vi "canDataSort.vi"() -> ()   [LabVIEW 2023] (continued)
      2032  1FFFFFFF   00000004    8        00\t00\tFF\tFF\tFF\tFF\tFF\tFF\r\n      2023  0CF102A7   00000004    8        30\t75\tE0\t2E\t80\tFF\tFF\tFD\r\n      2023  0CF101A7   00000004    8        68\t00\t97\tCC\t00\t16\t39\t7F\r\n      2046  18F121F0   00000004    8        09\t19\t00\t00\tFF\tFF\tB0\t01\r\n      2045  18F106A7   00000004    8        00\tF7\tFF\tFF\tFF\tFF\tFF\t99\r\n      2045  0CF104A7   00000004    8        F0\t60\t22\tFC\tFF\tFF\tFF\t4C\r\n      2044  0CF103A7   00000004    8        17\t1F\t08\t60\tB1\t1F\t08\t4C\r\n      2044  0CF102A7   00000004    8        30\t75\tE0\t2E\t80\tFF\tFF\tFD\r\n      2043  0C3C4D4A   00000004    8        BE\tFF\tFF\t7F\t18\tFF\tFF\t4C\r\n      2043  0CF101A7   00000004    8        68\t00\t97\tCC\t00\t16\t39\t80\r\n      2042  18F120F0   00000004    8        2B\t75\t60\tB1\tB0\t01\tFF\tFF\r\n      2041  18F11FF0   00000004    8        FF\t3F\t90\t68\t88\t1B\t10\tCC\r\n      2032  1FFFFFFF   00000004    8        00\t00\tFF\tFF\tFF\tFF\tFF\tFF\r\n      2023  0CF102A7   00000004    8        30\t75\tE0\t2E\t80\tFF\tFF\tFD\r\n      2047  1FFFFFFF   00000004    8        00\t00\tFF\tFF\tFF\tFF\tFF\tFF\r\n      2046  18F121F0   00000004    8        09\t19\t00\t00\tFF\tFF\tB0\t01\r\n      2045  18F106A7   00000004    8        00\tF7\tFF\tFF\tFF\tFF\tFF\t99\r\n      2045  0CF104A7   00000004    8        F0\t60\t22\tFC\tFF\tFF\tFF\t4C\r\n      2044  0CF103A7   00000004    8        17\t1F\t08\t60\tB1\t1F\t08\t4C\r\n      2044  0CF102A7   00000004    8        30\t75\tE0\t2E\t80\tFF\tFF\tFD\r\n      2043  0C3C4D4A   00000004    8        BE\tFF\tFF\t7F\t18\tFF\tFF\t4C\r\n      2043  0CF101A7   00000004    8        68\t00\t97\tCC\t00\t16\t39\t80\r\n      2042  18F120F0   00000004    8        2B\t75\t60\tB1\tB0\t01\tFF\tFF\r\n      2041  18F11FF0   00000004    8        FF\t3F\t90\t68\t88\t1B\t10\tCC\r\n      2032  1FFFFFFF   00000004    8        00\t00\tFF\tFF\tFF\tFF\tFF\tFF\r\n      2052  1FFFFFFF   00000004    8        00\t00\tFF\tFF\tFF\tFF\tFF\tFF\r\n      2047  1FFFFFFF   00000004    8        00\t00\tFF\tFF\tFF\tFF\tFF\tFF\r\n      2046  18F121F0   00000004    8        09\t19\t00\t00\tFF\tFF\tB0\t01\r\n      2045  18F106A7   00000004    8        00\tF7\tFF\tFF\tFF\tFF\tFF\t99\r\n      2045  0CF104A7   00000004    8        F0\t60\t22\tFC\tFF\tFF\tFF\t4C\r\n      2044  0CF103A7   00000004    8        17\t1F\t08\t60\tB1\t1F\t08\t4C\r\n      2044  0CF102A7   00000004    8        30\t75\tE0\t2E\t80\tFF\tFF\tFD\r\n      2043  0C3C4D4A   00000004    8        BE\tFF\tFF\t7F\t18\tFF\tFF\t4C\r\n      2043  0CF101A7   00000004    8        68\t00\t97\tCC\t00\t16\t39\t80\r\n      2042  18F120F0   00000004    8        2B\t75\t60\tB1\tB0\t01\tFF\tFF\r\n      2041  18F11FF0   00000004    8        FF\t3F\t90\t68\t88\t1B\t10\tCC\r\n      2062  1FFFFFFF   00000004    8        00\t00\tFF\tFF\tFF\tFF\tFF\tFF\r\n      2052  1FFFFFFF   00000004    8        00\t00\tFF\tFF\tFF\tFF\tFF\tFF\r\n      2047  1FFFFFFF   00000004    8        00\t00\tFF\tFF\tFF\tFF\tFF\tFF\r\n      2046  18F121F0   00000004    8        09\t19\t00\t00\tFF\tFF\tB0\t01\r\n      2045  18F106A7   00000004    8        00\tF7\tFF\tFF\tFF\tFF\tFF\t99\r\n      2045  0CF104A7   00000004    8        F0\t60\t22\tFC\tFF\tFF\tFF\t4C\r\n      2044  0CF103A7   00000004    8        17\t1F\t08\t60\tB1\t1F\t08\t4C\r\n      2044  0CF102A7   00000004    8        30\t75\tE0\t2E\t80\tFF\tFF\tFD\r\n      2043  0C3C4D4A   00000004    8        BE\tFF\tFF\t7F\t18\tFF\tFF\t4C\r\n      2043  0CF101A7   00000004    8        68\t00\t97\tCC\t00\t16\t39\t80\r\n      2042  18F120F0   00000004    8        2B\t75\t60\tB1\tB0\t01\tFF\tFF\r\n      2063  0CF101A7   00000004    8        68\t00\t97\tCC\t00\t16\t39\t81\r\n      2062  1FFFFFFF   00000004    8        00\t00\tFF\tFF\tFF\tFF\tFF\tFF\r\n      2052  1FFFFFFF   00000004    8        00\t00\tFF\tFF\tFF\tFF\tFF\tFF\r\n      2047  1FFFFFFF   00000004    8        00\t00\tFF\tFF\tFF\tFF\tFF\tFF\r\n      2046  18F121F0   00000004    8        09\t19\t00\t00\tFF\tFF\tB0\t01\r\n      2045  18F106A7   00000004    8        00\tF7\tFF\tFF\tFF\tFF\tFF\t99\r\n      2045  0CF104A7   00000004    8        F0\t60\t22\tFC\tFF\tFF\tFF\t4C\r\n      2044  0CF103A7   00000004    8        17\t1F\t08\t60\tB1\t1F\t08\t4C\r\n      2044  0CF102A7   00000004    8        30\t75\tE0\t2E\t80\tFF\tFF\tFD\r\n      2043  0C3C4D4A   00000004    8        BE\tFF\tFF\t7F\t18\tFF\tFF\t4C\r\n      2043  0CF101A7   00000004    8        68\t00\t97\tCC\t00\t16\t39\t80\r\n      2063  0CF102A7   00000004    8        30\t75\tE0\t2E\t80\tFF\tFF\tFD\r\n      2063  0CF101A7   00000004    8        68\t00\t97\tCC\t00\t16\t39\t81\r\n      2062  1FFFFFFF   00000004    8        00\t00\tFF\tFF\tFF\tFF\tFF\tFF\r\n      2052  1FFFFFFF   00000004    8        00\t00\tFF\tFF\tFF\tFF\tFF\tFF\r\n      2047  1FFFFFFF   00000004    8        00\t00\tFF\tFF\tFF\tFF\tFF\tFF\r\n      2046  18F121F0   00000004    8        09\t19\t00\t00\tFF\tFF\tB0\t01\r\n      2045  18F106A7   00000004    8        00\tF7\tFF\tFF\tFF\tFF\tFF\t99\r\n      2045  0CF104A7   00000004    8        F0\t60\t22\tFC\tFF\tFF\tFF\t4C\r\n      2044  0CF103A7   00000004    8        17\t1F\t08\t60\tB1\t1F\t08\t4C\r\n      2044  0CF102A7   00000004    8        30\t75\tE0\t2E\t80\tFF\tFF\tFD\r\n      2043  0C3C4D4A   00000004    8        BE\tFF\tFF\t7F\t18\tFF\tFF\t4C\r\n      2072  1FFFFFFF   00000004    8        00\t00\tFF\tFF\tFF\tFF\tFF\tFF\r\n      2063  0CF102A7   00000004    8        30\t75\tE0\t2E\t80\tFF\tFF\tFD\r\n      2063  0CF101A7   00000004    8        68\t00\t97\tCC\t00\t16\t39\t81\r\n      2062  1FFFFFFF   00000004    8        00\t00\tFF\tFF\tFF\tFF\tFF\tFF\r\n      2052  1FFFFFFF   00000004    8        00\t00\tFF\tFF\tFF\tFF\tFF\tFF\r\n      2047  1FFFFFFF   00000004    8        00\t00\tFF\tFF\tFF\tFF\tFF\tFF\r\n      2046  18F121F0   00000004    8        09\t19\t00\t00\tFF\tFF\tB0\t01\r\n      2045  18F106A7   00000004    8        00\tF7\tFF\tFF\tFF\tFF\tFF\t99\r\n      2045  0CF104A7   00000004    8        F0\t60\t22\tFC\tFF\tFF\tFF\t4C\r\n      2044  0CF103A7   00000004    8        17\t1F\t08\t60\tB1\t1F\t08\t4C\r\n      2044  0CF102A7   00000004    8        30\t75\tE0\t2E\t80\tFF\tFF\tFD\r\n      2082  1FFFFFFF   00000004    8        00\t00\tFF\tFF\tFF\tFF\tFF\tFF\r\n      2072  1FFFFFFF   00000004    8        00\t00\tFF\tFF\tFF\tFF\tFF\tFF\r\n      2063  0CF102A7   00000004    8        30\t75\tE0\t2E\t80\tFF\tFF\tFD\r\n      2063  0CF101A7   00000004    8        68\t00\t97\tCC\t00\t16\t39\t81\r\n      2062  1FFFFFFF   00000004    8        00\t00\tFF\tFF\tFF\tFF\tFF\tFF\r\n      2052  1FFFFFFF   00000004    8        00\t00\tFF\tFF\tFF\tFF\tFF\tFF\r\n      2047  1FFFFFFF   00000004    8        00\t00\tFF\tFF\tFF\tFF\tFF\tFF\r\n      2046  18F121F0   00000004    8        09\t19\t00\t00\tFF\tFF\tB0\t01\r\n      2045  18F106A7   00000004    8        00\tF7\tFF\tFF\tFF\tFF\tFF\t99\r\n      2045  0CF104A7   00000004    8        F0\t60\t22\tFC\tFF\tFF\tFF\t4C\r\n      2044  0CF103A7   00000004    8        17\t1F\t08\t60\tB1\t1F\t08\t4C\r\n      2083  0CF101A7   00000004    8        68\t00\t97\tCC\t00\t16\t39\t82\r\n      2082  1FFFFFFF   00000004    8        00\t00\tFF\tFF\tFF\tFF\tFF\tFF\r\n      2072  1FFFFFFF   00000004    8        00\t00\tFF\tFF\tFF\tFF\tFF\tFF\r\n      2063  0CF102A7   00000004    8        30\t75\tE0\t2E\t80\tFF\tFF\tFD\r\n      2063  0CF101A7   00000004    8        68\t00\t97\tCC\t00\t16\t39\t81\r\n      2062  1FFFFFFF   00000004    8        00\t00\tFF\tFF\tFF\tFF\tFF\tFF\r\n      2052  1FFFFFFF   00000004    8        00\t00\tFF\tFF\tFF\tFF\tFF\tFF\r\n      2047  1FFFFFFF   00000004    8        00\t00\tFF\tFF\tFF\tFF\tFF\tFF\r\n      2046  18F121F0   00000004    8        09\t19\t00\t00\tFF\tFF\tB0\t01\r\n      2045  18F106A7   00000004    8        00\tF7\tFF\tFF\tFF\tFF\tFF\t99\r\n      2045  0CF104A7   00000004    8        F0\t60\t22\tFC\tFF\tFF\tFF\t4C\r\n      2083  0CF102A7   00000004    8        30\t75\tE0\t2E\t80\tFF\tFF\tFD\r\n      2083  0CF101A7   00000004    8        68\t00\t97\tCC\t00\t16\t39\t82\r\n      2082  1FFFFFFF   00000004    8        00\t00\tFF\tFF\tFF\tFF\tFF\tFF\r\n      2072  1FFFFFFF   00000004    8        00\t00\tFF\tFF\tFF\tFF\tFF\tFF\r\n      2063  0CF102A7   00000004    8        30\t75\tE0\t2E\t80\tFF\tFF\tFD\r\n      2063  0CF101A7   00000004    8        68\t00\t97\tCC\t00\t16\t39\t81\r\n      2062  1FFFFFFF   00000004    8        00\t00\tFF\tFF\tFF\tFF\tFF\tFF\r\n      2052  1FFFFFFF   00000004    8        00\t00\tFF\tFF\tFF\tFF\tFF\tFF\r\n      2047  1FFFFFFF   00000004    8        00\t00\tFF\tFF\tFF\tFF\tFF\tFF\r\n      2046  18F121F0   00000004    8        09\t19\t00\t00\tFF\tFF\tB0\t01\r\n      2045  18F106A7   00000004    8        00\tF7\tFF\tFF\tFF\tFF\tFF\t99\r\n      2092  1FFFFFFF   00000004    8        00\t00\tFF\tFF\tFF\tFF\tFF\tFF\r\n      2083  0CF102A7   00000004    8        30\t75\tE0\t2E\t80\tFF\tFF\tFD\r\n      2083  0CF101A7   00000004    8        68\t00\t97\tCC\t00\t16\t39\t82\r\n      2082  1FFFFFFF   00000004    8        00\t00\tFF\tFF\tFF\tFF\tFF\tFF\r\n      2072  1FFFFFFF   00000004    8        00\t00\tFF\tFF\tFF\tFF\tFF\tFF\r\n      2063  0CF102A7   00000004    8        30\t75\tE0\t2E\t80\tFF\tFF\tFD\r\n      2063  0CF101A7   00000004    8        68\t00\t97\tCC\t00\t16\t39\t81\r\n      2062  1FFFFFFF   00000004    8        00\t00\tFF\tFF\tFF\tFF\tFF\tFF\r\n      2052  1FFFFFFF   00000004    8        00\t00\tFF\tFF\tFF\tFF\tFF\tFF\r\n      2047  1FFFFFFF   00000004    8        00\t00\tFF\tFF\tFF\tFF\tFF\tFF\r\n      2046  18F121F0   00000004    8        09\t19\t00\t00\tFF\tFF\tB0\t01\r\n      2093  18F106A7   00000004    8        00\tF7\tFF\tFF\tFF\tFF\tFF\t9A\r\n      2092  1FFFFFFF   00000004    8        00\t00\tFF\tFF\tFF\tFF\tFF\tFF\r\n      2083  0CF102A7   00000004    8        30\t75\tE0\t2E\t80\tFF\tFF\tFD\r\n      2083  0CF101A7   00000004    8        68\t00\t97\tCC\t00\t16\t39\t82\r\n      2082  1FFFFFFF   00000004    8        00\t00\tFF\tFF\tFF\tFF\tFF\tFF\r\n      2072  1FFFFFFF   00000004    8        00\t00\tFF\tFF\tFF\tFF\tFF\tFF\r\n      2063  0CF102A7   00000004    8        30\t75\tE0\t2E\t80\tFF\tFF\tFD\r\n      2063  0CF101A7   00000004    8        68\t00\t97\tCC\t00\t16\t39\t81\r\n      2062  1FFFFFFF   00000004    8        00\t00\tFF\tFF\tFF\tFF\tFF\tFF\r\n      2052  1FFFFFFF   00000004    8        00\t00\tFF\tFF\tFF\tFF\tFF\tFF\r\n      2047  1FFFFFFF   00000004    8        00\t00\tFF\tFF\tFF\tFF\tFF\tFF\r\n      2102  1FFFFFFF   00000004    8        00\t00\tFF\tFF\tFF\tFF\tFF\tFF\r\n      2093  18F106A7   00000004    8        00\tF7\tFF\tFF\tFF\tFF\tFF\t9A\r\n      2092  1FFFFFFF   00000004    8        00\t00\tFF\tFF\tFF\tFF\tFF\tFF\r\n      2083  0CF102A7   00000004    8        30\t75\tE0\t2E\t80\tFF\tFF\tFD\r\n      2083  0CF101A7   00000004    8        68\t00\t97\tCC\t00\t16\t39\t82\r\n      2082  1FFFFFFF   00000004    8        00\t00\tFF\tFF\tFF\tFF\tFF\tFF\r\n      2072  1FFFFFFF   00000004    8        00\t00\tFF\tFF\tFF\tFF\tFF\tFF\r\n      2063  0CF102A7   00000004    8        30\t75\tE0\t2E\t80\tFF\tFF\tFD\r\n      2063  0CF101A7   00000004    8        68\t00\t97\tCC\t00\t16\t39\t81\r\n      2062  1FFFFFFF   00000004    8        00\t00\tFF\tFF\tFF\tFF\tFF\tFF\r\n      2052  1FFFFFFF   00000004    8        00\t00\tFF\tFF\tFF\tFF\tFF\tFF\r\n      2103  0CF101A7   00000004    8        68\t00\t97\tCC\t00\t16\t39\t83\r\n      2102  1FFFFFFF   00000004    8        00\t00\tFF\tFF\tFF\tFF\tFF\tFF\r\n      2093  18F106A7   00000004    8        00\tF7\tFF\tFF\tFF\tFF\tFF\t9A\r\n      2092  1FFFFFFF   00000004    8        00\t00\tFF\tFF\tFF\tFF\tFF\tFF\r\n      2083  0CF102A7   00000004    8        30\t75\tE0\t2E\t80\tFF\tFF\tFD\r\n      2083  0CF101A7   00000004    8        68\t00\t97\tCC\t00\t16\t39\t82\r\n      2082  1FFFFFFF   00000004    8        00\t00\tFF\tFF\tFF\tFF\tFF\tFF\r\n      2072  1FFFFFFF   00000004    8        00\t00\tFF\tFF\tFF\tFF\tFF\tFF\r\n      2063  0CF102A7   00000004    8        30\t75\tE0\t2E\t80\tFF\tFF\tFD\r\n      2063  0CF101A7   00000004    8        68\t00\t97\tCC\t00\t16\t39\t81\r\n      2062  1FFFFFFF   00000004    8        00\t00\tFF\tFF\tFF\tFF\tFF\tFF\r\n      2103  0CF102A7   00000004    8        30\t75\tE0\t2E\t80\tFF\tFF\tFD\r\n      2103  0CF101A7   00000004    8        68\t00\t97\tCC\t00\t16\t39\t83\r\n      2102  1FFFFFFF   00000004    8        00\t00\tFF\tFF\tFF\tFF\tFF\tFF\r\n      2093  18F106A7   00000004    8        00\tF7\tFF\tFF\tFF\tFF\tFF\t9A\r\n      2092  1FFFFFFF   00000004    8        00\t00\tFF\tFF\tFF\tFF\tFF\tFF\r\n      2083  0CF102A7   00000004    8        30\t75\tE0\t2E\t80\tFF\tFF\tFD\r\n      2083  0CF101A7   00000004    8        68\t00\t97\tCC\t00\t16\t39\t82\r\n      2082  1FFFFFFF   00000004    8        00\t00\tFF\tFF\tFF\tFF\tFF\tFF\r\n      2072  1FFFFFFF   00000004    8        00\t00\tFF\tFF\tFF\tFF\tFF\tFF\r\n      2063  0CF102A7   00000004    8        30\t75\tE0\t2E\t80\tFF\tFF\tFD\r\n      2063  0CF101A7   00000004    8        68\t00\t97\tCC\t00\t16\t39\t81\r\n      2112  1FFFFFFF   00000004    8        00\t00\tFF\tFF\tFF\tFF\tFF\tFF\r\n      2103  0CF102A7   00000004    8        30\t75\tE0\t2E\t80\tFF\tFF\tFD\r\n      2103  0CF101A7   00000004    8        68\t00\t97\tCC\t00\t16\t39\t83\r\n      2102  1FFFFFFF   00000004    8        00\t00\tFF\tFF\tFF\tFF\tFF\tFF\r\n      2093  18F106A7   00000004    8        00\tF7\tFF\tFF\tFF\tFF\tFF\t9A\r\n      2092  1FFFFFFF   00000004    8        00\t00\tFF\tFF\tFF\tFF\tFF\tFF\r\n      2083  0CF102A7   00000004    8        30\t75\tE0\t2E\t80\tFF\tFF\tFD\r\n      2083  0CF101A7   00000004    8        68\t00\t97\tCC\t00\t16\t39\t82\r\n      2082  1FFFFFFF   00000004    8        00\t00\tFF\tFF\tFF\tFF\tFF\tFF\r\n      2072  1FFFFFFF   00000004    8        00\t00\tFF\tFF\tFF\tFF\tFF\tFF\r\n      2063  0CF102A7   00000004    8        30\t75\tE0\t2E\t80\tFF\tFF\tFD\r\n      2122  1FFFFFFF   00000004    8        00\t00\tFF\tFF\tFF\tFF\tFF\tFF\r\n      2112  1FFFFFFF   00000004    8        00\t00\tFF\tFF\tFF\tFF\tFF\tFF\r\n      2103  0CF102A7   00000004    8        30\t75\tE0\t2E\t80\tFF\tFF\tFD\r\n      2103  0CF101A7   00000004    8        68\t00\t97\tCC\t00\t16\t39\t83\r\n      2102  1FFFFFFF   00000004    8        00\t00\tFF\tFF\tFF\tFF\tFF\tFF\r\n      2093  18F106A7   00000004    8        00\tF7\tFF\tFF\tFF\tFF\tFF\t9A\r\n      2092  1FFFFFFF   00000004    8        00\t00\tFF\tFF\tFF\tFF\tFF\tFF\r\n      2083  0CF102A7   00000004    8        30\t75\tE0\t2E\t80\tFF\tFF\tFD\r\n      2083  0CF101A7   00000004    8        68\t00\t97\tCC\t00\t16\t39\t82\r\n      2082  1FFFFFFF   00000004    8        00\t00\tFF\tFF\tFF\tFF\tFF\tFF\r\n      2072  1FFFFFFF   00000004    8        00\t00\tFF\tFF\tFF\tFF\tFF\tFF\r\n      2123  0CF101A7   00000004    8        68\t00\t97\tCC\t00\t16\t39\t84\r\n      2122  1FFFFFFF   00000004    8        00\t00\tFF\tFF\tFF\tFF\tFF\tFF\r\n      2112  1FFFFFFF   00000004    8        00\t00\tFF\tFF\tFF\tFF\tFF\tFF\r\n      2103  0CF102A7   00000004    8        30\t75\tE0\t2E\t80\tFF\tFF\tFD\r\n      2103  0CF101A7   00000004    8        68\t00\t97\tCC\t00\t16\t39\t83\r\n      2102  1FFFFFFF   00000004    8        00\t00\tFF\tFF\tFF\tFF\tFF\tFF\r\n      2093  18F106A7   00000004    8        00\tF7\tFF\tFF\tFF\tFF\tFF\t9A\r\n      2092  1FFFFFFF   00000004    8        00\t00\tFF\tFF\tFF\tFF\tFF\tFF\r\n      2083  0CF102A7   00000004    8        30\t75\tE0\t2E\t80\tFF\tFF\tFD\r\n      2083  0CF101A7   00000004    8        68\t00\t97\tCC\t00\t16\t39\t82\r\n      2082  1FFFFFFF   00000004    8        00\t00\tFF\tFF\tFF\tFF\tFF\tFF\r\n      2123  0CF102A7   00000004    8        30\t75\tE0\t2E\t80\tFF\tFF\tFD\r\n      2123  0CF101A7   00000004    8        68\t00\t97\tCC\t00\t16\t39\t84\r\n      2122  1FFFFFFF   00000004    8        00\t00\tFF\tFF\tFF\tFF\tFF\tFF\r\n      2112  1FFFFFFF   00000004    8        00\t00\tFF\tFF\tFF\tFF\tFF\tFF\r\n      2103  0CF102A7   00000004    8        30\t75\tE0\t2E\t80\tFF\tFF\tFD\r\n      2103  0CF101A7   00000004    8        68\t00\t97\tCC\t00\t16\t39\t83\r\n      2102  1FFFFFFF   00000004    8        00\t00\tFF\tFF\tFF\tFF\tFF\tFF\r\n      2093  18F106A7   00000004    8        00\tF7\tFF\tFF\tFF\tFF\tFF\t9A\r\n      2092  1FFFFFFF   00000004    8        00\t00\tFF\tFF\tFF\tFF\tFF\tFF\r\n      2083  0CF102A7   00000004    8        30\t75\tE0\t2E\t80\tFF\tFF\tFD\r\n      2083  0CF101A7   00000004    8        68\t00\t97\tCC\t00\t16\t39\t82\r\n      2132  1FFFFFFF   00000004    8        00\t00\tFF\tFF\tFF\tFF\tFF\tFF\r\n      2123  0CF102A7   00000004    8        30\t75\tE0\t2E\t80\tFF\tFF\tFD\r\n      2123  0CF101A7   00000004    8        68\t00\t97\tCC\t00\t16\t39\t84\r\n      2122  1FFFFFFF   00000004    8        00\t00\tFF\tFF\tFF\tFF\tFF\tFF\r\n      2112  1FFFFFFF   00000004    8        00\t00\tFF\tFF\tFF\tFF\tFF\tFF\r\n      2103  0CF102A7   00000004    8        30\t75\tE0\t2E\t80\tFF\tFF\tFD\r\n      2103  0CF101A7   00000004    8        68\t00\t97\tCC\t00\t16\t39\t83\r\n      2102  1FFFFFFF   00000004    8        00\t00\tFF\tFF\tFF\tFF\tFF\tFF\r\n      2093  18F106A7   00000004    8        00\tF7\tFF\tFF\tFF\tFF\tFF\t9A\r\n      2092  1FFFFFFF   00000004    8        00\t00\tFF\tFF\tFF\tFF\tFF\tFF\r\n      2083  0CF102A7   00000004    8        30\t75\tE0\t2E\t80\tFF\tFF\tFD\r\n      2141  18F11FF0   00000004    8        FF\t3F\t90\t68\t88\t1B\t10\tDC\r\n      2132  1FFFFFFF   00000004    8        00\t00\tFF\tFF\tFF\tFF\tFF\tFF\r\n      2123  0CF102A7   00000004    8        30\t75\tE0\t2E\t80\tFF\tFF\tFD\r\n      2123  0CF101A7   00000004    8        68\t00\t97\tCC\t00\t16\t39\t84\r\n      2122  1FFFFFFF   00000004    8        00\t00\tFF\tFF\tFF\tFF\tFF\tFF\r\n      2112  1FFFFFFF   00000004    8        00\t00\tFF\tFF\tFF\tFF\tFF\tFF\r\n      2103  0CF102A7   00000004    8        30\t75\tE0\t2E\t80\tFF\tFF\tFD\r\n      2103  0CF101A7   00000004    8        68\t00\t97\tCC\t00\t16\t39\t83\r\n      2102  1FFFFFFF   00000004    8        00\t00\tFF\tFF\tFF\tFF\tFF\tFF\r\n      2093  18F106A7   00000004    8        00\tF7\tFF\tFF\tFF\tFF\tFF\t9A\r\n      2092  1FFFFFFF   00000004    8        00\t00\tFF\tFF\tFF\tFF\tFF\tFF\r\n      2142  18F120F0   00000004    8        2B\t75\t60\tB1\tB0\t01\tFF\tFF\r\n      2141  18F11FF0   00000004    8        FF\t3F\t90\t68\t88\t1B\t10\tDC\r\n      2132  1FFFFFFF   00000004    8        00\t00\tFF\tFF\tFF\tFF\tFF\tFF\r\n      2123  0CF102A7   00000004    8        30\t75\tE0\t2E\t80\tFF\tFF\tFD\r\n      2123  0CF101A7   00000004    8        68\t00\t97\tCC\t00\t16\t39\t84\r\n      2122  1FFFFFFF   00000004    8        00\t00\tFF\tFF\tFF\tFF\tFF\tFF\r\n      2112  1FFFFFFF   00000004    8        00\t00\tFF\tFF\tFF\tFF\tFF\tFF\r\n      2103  0CF102A7   00000004    8        30\t75\tE0\t2E\t80\tFF\tFF\tFD\r\n      2103  0CF101A7   00000004    8        68\t00\t97\tCC\t00\t16\t39\t83\r\n      2102  1FFFFFFF   00000004    8        00\t00\tFF\tFF\tFF\tFF\tFF\tFF\r\n      2093  18F106A7   00000004    8        00\tF7\tFF\tFF\tFF\tFF\tFF\t9A\r\n      2143  0CF101A7   00000004    8        68\t00\t97\tCC\t00\t16\t39\t85\r\n      2142  18F120F0   00000004    8        2B\t75\t60\tB1\tB0\t01\tFF\tFF\r\n      2141  18F11FF0   00000004    8        FF\t3F\t90\t68\t88\t1B\t10\tDC\r\n      2132  1FFFFFFF   00000004    8        00\t00\tFF\tFF\tFF\tFF\tFF\tFF\r\n      2123  0CF102A7   00000004    8        30\t75\tE0\t2E\t80\tFF\tFF\tFD\r\n      2123  0CF101A7   00000004    8        68\t00\t97\tCC\t00\t16\t39\t84\r\n      2122  1FFFFFFF   00000004    8        00\t00\tFF\tFF\tFF\tFF\tFF\tFF\r\n      2112  1FFFFFFF   00000004    8        00\t00\tFF\tFF\tFF\tFF\tFF\tFF\r\n      2103  0CF102A7   00000004    8        30\t75\tE0\t2E\t80\tFF\tFF\tFD\r\n      2103  0CF101A7   00000004    8        68\t00\t97\tCC\t00\t16\t39\t83\r\n      2102  1FFFFFFF   00000004    8        00\t00\tFF\tFF\tFF\tFF\tFF\tFF\r\n      2143  0CF102A7   00000004    8        30\t75\tE0\t2E\t80\tFF\tFF\tFD\r\n      2143  0CF101A7   00000004    8        68\t00\t97\tCC\t00\t16\t39\t85\r\n      2142  18F120F0   00000004    8        2B\t75\t60\tB1\tB0\t01\tFF\tFF\r\n      2141  18F11FF0   00000004    8        FF\t3F\t90\t68\t88\t1B\t10\tDC\r\n      2132  1FFFFFFF   00000004    8        00\t00\tFF\tFF\tFF\tFF\tFF\tFF\r\n      2123  0CF102A7   00000004    8        30\t75\tE0\t2E\t80\tFF\tFF\tFD\r\n      2123  0CF101A7   00000004    8        68\t00\t97\tCC\t00\t16\t39\t84\r\n      2122  1FFFFFFF   00000004    8        00\t00\tFF\tFF\tFF\tFF\tFF\tFF\r\n      2112  1FFFFFFF   00000004    8        00\t00\tFF\tFF\tFF\tFF\tFF\tFF\r\n      2103  0CF102A7   00000004    8        30\t75\tE0\t2E\t80\tFF\tFF\tFD\r\n      2103  0CF101A7   00000004    8        68\t00\t97\tCC\t00\t16\t39\t83\r\n      2144  0C3C4D4A   00000004    8        BE\tFF\tFF\t7F\t18\tFF\tFF\t4D\r\n      2143  0CF102A7   00000004    8        30\t75\tE0\t2E\t80\tFF\tFF\tFD\r\n      2143  0CF101A7   00000004    8        68\t00\t97\tCC\t00\t16\t39\t85\r\n      2142  18F120F0   00000004    8        2B\t75\t60\tB1\tB0\t01\tFF\tFF\r\n      2141  18F11FF0   00000004    8        FF\t3F\t90\t68\t88\t1B\t10\tDC\r\n      2132  1FFFFFFF   00000004    8        00\t00\tFF\tFF\tFF\tFF\tFF\tFF\r\n      2123  0CF102A7   00000004    8        30\t75\tE0\t2E\t80\tFF\tFF\tFD\r\n      2123  0CF101A7   00000004    8        68\t00\t97\tCC\t00\t16\t39\t84\r\n      2122  1FFFFFFF   00000004    8        00\t00\tFF\tFF\tFF\tFF\tFF\tFF\r\n      2112  1FFFFFFF   00000004    8        00\t00\tFF\tFF\tFF\tFF\tFF\tFF\r\n      2103  0CF102A7   00000004    8        30\t75\tE0\t2E\t80\tFF\tFF\tFD\r\n      2144  0CF103A7   00000004    8        17\t1F\t08\t60\tB1\t1F\t08\t4D\r\n      2144  0C3C4D4A   00000004    8        BE\tFF\tFF\t7F\t18\tFF\tFF\t4D\r\n      2143  0CF102A7   00000004    8        30\t75\tE0\t2E\t80\tFF\tFF\tFD\r\n      2143  0CF101A7   00000004    8        68\t00\t97\tCC\t00\t16\t39\t85\r\n      2142  18F120F0   00000004    8        2B\t75\t60\tB1\tB0\t01\tFF\tFF\r\n      2141  18F11FF0   00000004    8        FF\t3F\t90\t68\t88\t1B\t10\tDC\r\n      2132  1FFFFFFF   00000004    8        00\t00\tFF\tFF\tFF\tFF\tFF\tFF\r\n      2123  0CF102A7   00000004    8        30\t75\tE0\t2E\t80\tFF\tFF\tFD\r\n      2123  0CF101A7   00000004    8        68\t00\t97\tCC\t00\t16\t39\t84\r\n      2122  1FFFFFFF   00000004    8        00\t00\tFF\tFF\tFF\tFF\tFF\tFF\r\n      2112  1FFFFFFF   00000004    8        00\t00\tFF\tFF\tFF\tFF\tFF\tFF\r\n      2145  0CF104A7   00000004    8        F0\t60\t22\tFC\tFF\tFF\tFF\t4D\r\n      2144  0CF103A7   00000004    8        17\t1F\t08\t60\tB1\t1F\t08\t4D\r\n      2144  0C3C4D4A   00000004    8        BE\tFF\tFF\t7F\t18\tFF\tFF\t4D\r\n      2143  0CF102A7   00000004    8        30\t75\tE0\t2E\t80\tFF\tFF\tFD\r\n      2143  0CF101A7   00000004    8        68\t00\t97\tCC\t00\t16\t39\t85\r\n      2142  18F120F0   00000004    8        2B\t75\t60\tB1\tB0\t01\tFF\tFF\r\n      2141  18F11FF0   00000004    8        FF\t3F\t90\t68\t88\t1B\t10\tDC\r\n      2132  1FFFFFFF   00000004    8        00\t00\tFF\tFF\tFF\tFF\tFF\tFF\r\n      2123  0CF102A7   00000004    8        30\t75\tE0\t2E\t80\tFF\tFF\tFD\r\n      2123  0CF101A7   00000004    8        68\t00\t97\tCC\t00\t16\t39\t84\r\n      2122  1FFFFFFF   00000004    8        00\t00\tFF\tFF\tFF\tFF\tFF\tFF\r\n      2145  18F106A7   00000004    8        00\tF7\tFF\tFF\tFF\tFF\tFF\t9B\r\n      2145  0CF104A7   00000004    8        F0\t60\t22\tFC\tFF\tFF\tFF\t4D\r\n      2144  0CF103A7   00000004    8        17\t1F\t08\t60\tB1\t1F\t08\t4D\r\n      2144  0C3C4D4A   00000004    8        BE\tFF\tFF\t7F\t18\tFF\tFF\t4D\r\n      2143  0CF102A7   00000004    8        30\t75\tE0\t2E\t80\tFF\tFF\tFD\r\n      2143  0CF101A7   00000004    8        68\t00\t97\tCC\t00\t16\t39\t85\r\n      2142  18F120F0   00000004    8        2B\t75\t60\tB1\tB0\t01\tFF\tFF\r\n      2141  18F11FF0   00000004    8        FF\t3F\t90\t68\t88\t1B\t10\tDC\r\n      2132  1FFFFFFF   00000004    8        00\t00\tFF\tFF\tFF\tFF\tFF\tFF\r\n      2123  0CF102A7   00000004    8        30\t75\tE0\t2E\t80\tFF\tFF\tFD\r\n      2123  0CF101A7   00000004    8        68\t00\t97\tCC\t00\t16\t39\t84\r\n      2146  18F108A7   00000004    8        F0\t00\t00\tFF\tFF\tFF\tFF\t42\r\n      2145  18F106A7   00000004    8        00\tF7\tFF\tFF\tFF\tFF\tFF\t9B\r\n      2145  0CF104A7   00000004    8        F0\t60\t22\tFC\tFF\tFF\tFF\t4D\r\n      2144  0CF103A7   00000004    8        17\t1F\t08\t60\tB1\t1F\t08\t4D\r\n      2144  0C3C4D4A   00000004    8        BE\tFF\tFF\t7F\t18\tFF\tFF\t4D\r\n      2143  0CF102A7   00000004    8        30\t75\tE0\t2E\t80\tFF\tFF\tFD\r\n      2143  0CF101A7   00000004    8        68\t00\t97\tCC\t00\t16\t39\t85\r\n      2142  18F120F0   00000004    8        2B\t75\t60\tB1\tB0\t01\tFF\tFF\r\n      2141  18F11FF0   00000004    8        FF\t3F\t90\t68\t88\t1B\t10\tDC\r\n      2132  1FFFFFFF   00000004    8        00\t00\tFF\tFF\tFF\tFF\tFF\tFF\r\n      2123  0CF102A7   00000004    8        30\t75\tE0\t2E\t80\tFF\tFF\tFD\r\n      2146  18F121F0   00000004    8        09\t19\t00\t00\tFF\tFF\tB0\t01\r\n      2146  18F108A7   00000004    8        F0\t00\t00\tFF\tFF\tFF\tFF\t42\r\n      2145  18F106A7   00000004    8        00\tF7\tFF\tFF\tFF\tFF\tFF\t9B\r\n      2145  0CF104A7   00000004    8        F0\t60\t22\tFC\tFF\tFF\tFF\t4D\r\n      2144  0CF103A7   00000004    8        17\t1F\t08\t60\tB1\t1F\t08\t4D\r\n      2144  0C3C4D4A   00000004    8        BE\tFF\tFF\t7F\t18\tFF\tFF\t4D\r\n      2143  0CF102A7   00000004    8        30\t75\tE0\t2E\t80\tFF\tFF\tFD\r\n      2143  0CF101A7   00000004    8        68\t00\t97\tCC\t00\t16\t39\t85\r\n      2142  18F120F0   00000004    8        2B\t75\t60\tB1\tB0\t01\tFF\tFF\r\n      2141  18F11FF0   00000004    8        FF\t3F\t90\t68\t88\t1B\t10\tDC\r\n      2132  1FFFFFFF   00000004    8        00\t00\tFF\tFF\tFF\tFF\tFF\tFF\r\n      2147  18FEF117   00000004    8        F7\t97\tCC\tCF\tFF\tFF\tFF\tFF\r\n      2146  18F121F0   00000004    8        09\t19\t00\t00\tFF\tFF\tB0\t01\r\n      2146  18F108A7   00000004    8        F0\t00\t00\tFF\tFF\tFF\tFF\t42\r\n      2145  18F106A7   00000004    8        00\tF7\tFF\tFF\tFF\tFF\tFF\t9B\r\n      2145  0CF104A7   00000004    8        F0\t60\t22\tFC\tFF\tFF\tFF\t4D\r\n      2144  0CF103A7   00000004    8        17\t1F\t08\t60\tB1\t1F\t08\t4D\r\n      2144  0C3C4D4A   00000004    8        BE\tFF\tFF\t7F\t18\tFF\tFF\t4D\r\n      2143  0CF102A7   00000004    8        30\t75\tE0\t2E\t80\tFF\tFF\tFD\r\n      2143  0CF101A7   00000004    8        68\t00\t97\tCC\t00\t16\t39\t85\r\n      2142  18F120F0   00000004    8        2B\t75\t60\tB1\tB0\t01\tFF\tFF\r\n      2141  18F11FF0   00000004    8        FF\t3F\t90\t68\t88\t1B\t10\tDC\r\n      2148  1FFFFFFF   00000004    8        00\t00\tFF\tFF\tFF\tFF\tFF\tFF\r\n      2147  18FEF117   00000004    8        F7\t97\tCC\tCF\tFF\tFF\tFF\tFF\r\n      2146  18F121F0   00000004    8        09\t19\t00\t00\tFF\tFF\tB0\t01\r\n      2146  18F108A7   00000004    8        F0\t00\t00\tFF\tFF\tFF\tFF\t42\r\n      2145  18F106A7   00000004    8        00\tF7\tFF\tFF\tFF\tFF\tFF\t9B\r\n      2145  0CF104A7   00000004    8        F0\t60\t22\tFC\tFF\tFF\tFF\t4D\r\n      2144  0CF103A7   00000004    8        17\t1F\t08\t60\tB1\t1F\t08\t4D\r\n      2144  0C3C4D4A   00000004    8        BE\tFF\tFF\t7F\t18\tFF\tFF\t4D\r\n      2143  0CF102A7   00000004    8        30\t75\tE0\t2E\t80\tFF\tFF\tFD\r\n      2143  0CF101A7   00000004    8        68\t00\t97\tCC\t00\t16\t39\t85\r\n      2142  18F120F0   00000004    8        2B\t75\t60\tB1\tB0\t01\tFF\tFF\r\n      2152  1FFFFFFF   00000004    8        00\t00\tFF\tFF\tFF\tFF\tFF\tFF\r\n      2148  1FFFFFFF   00000004    8        00\t00\tFF\tFF\tFF\tFF\tFF\tFF\r\n      2147  18FEF117   00000004    8        F7\t97\tCC\tCF\tFF\tFF\tFF\tFF\r\n      2146  18F121F0   00000004    8        09\t19\t00\t00\tFF\tFF\tB0\t01\r\n      2146  18F108A7   00000004    8        F0\t00\t00\tFF\tFF\tFF\tFF\t42\r\n      2145  18F106A7   00000004    8        00\tF7\tFF\tFF\tFF\tFF\tFF\t9B\r\n      2145  0CF104A7   00000004    8        F0\t60\t22\tFC\tFF\tFF\tFF\t4D\r\n      2144  0CF103A7   00000004    8        17\t1F\t08\t60\tB1\t1F\t08\t4D\r\n      2144  0C3C4D4A   00000004    8        BE\tFF\tFF\t7F\t18\tFF\tFF\t4D\r\n      2143  0CF102A7   00000004    8        30\t75\tE0\t2E\t80\tFF\tFF\tFD\r\n      2143  0CF101A7   00000004    8        68\t00\t97\tCC\t00\t16\t39\t85\r\n      2162  1FFFFFFF   00000004    8        00\t00\tFF\tFF\tFF\tFF\tFF\tFF\r\n      2152  1FFFFFFF   00000004    8        00\t00\tFF\tFF\tFF\tFF\tFF\tFF\r\n      2148  1FFFFFFF   00000004    8        00\t00\tFF\tFF\tFF\tFF\tFF\tFF\r\n      2147  18FEF117   00000004    8        F7\t97\tCC\tCF\tFF\tFF\tFF\tFF\r\n      2146  18F121F0   00000004    8        09\t19\t00\t00\tFF\tFF\tB0\t01\r\n      2146  18F108A7   00000004    8        F0\t00\t00\tFF\tFF\tFF\tFF\t42\r\n      2145  18F106A7   00000004    8        00\tF7\tFF\tFF\tFF\tFF\tFF\t9B\r\n      2145  0CF104A7   00000004    8        F0\t60\t22\tFC\tFF\tFF\tFF\t4D\r\n      2144  0CF103A7   00000004    8        17\t1F\t08\t60\tB1\t1F\t08\t4D\r\n      2144  0C3C4D4A   00000004    8        BE\tFF\tFF\t7F\t18\tFF\tFF\t4D\r\n      2143  0CF102A7   00000004    8        30\t75\tE0\t2E\t80\tFF\tFF\tFD\r\n      2163  0CF101A7   00000004    8        68\t00\t97\tCC\t00\t16\t39\t86\r\n      2162  1FFFFFFF   00000004    8        00\t00\tFF\tFF\tFF\tFF\tFF\tFF\r\n      2152  1FFFFFFF   00000004    8        00\t00\tFF\tFF\tFF\tFF\tFF\tFF\r\n      2148  1FFFFFFF   00000004    8        00\t00\tFF\tFF\tFF\tFF\tFF\tFF\r\n      2147  18FEF117   00000004    8        F7\t97\tCC\tCF\tFF\tFF\tFF\tFF\r\n      2146  18F121F0   00000004    8        09\t19\t00\t00\tFF\tFF\tB0\t01\r\n      2146  18F108A7   00000004    8        F0\t00\t00\tFF\tFF\tFF\tFF\t42\r\n      2145  18F106A7   00000004    8        00\tF7\tFF\tFF\tFF\tFF\tFF\t9B\r\n      2145  0CF104A7   00000004    8        F0\t60\t22\tFC\tFF\tFF\tFF\t4D\r\n      2144  0CF103A7   00000004    8        17\t1F\t08\t60\tB1\t1F\t08\t4D\r\n      2144  0C3C4D4A   00000004    8        BE\tFF\tFF\t7F\t18\tFF\tFF\t4D\r\n      2163  0CF102A7   00000004    8        30\t75\tE0\t2E\t80\tFF\tFF\tFD\r\n      2163  0CF101A7   00000004    8        68\t00\t97\tCC\t00\t16\t39\t86\r\n      2162  1FFFFFFF   00000004    8        00\t00\tFF\tFF\tFF\tFF\tFF\tFF\r\n      2152  1FFFFFFF   00000004    8        00\t00\tFF\tFF\tFF\tFF\tFF\tFF\r\n      2148  1FFFFFFF   00000004    8        00\t00\tFF\tFF\tFF\tFF\tFF\tFF\r\n      2147  18FEF117   00000004    8        F7\t97\tCC\tCF\tFF\tFF\tFF\tFF\r\n      2146  18F121F0   00000004    8        09\t19\t00\t00\tFF\tFF\tB0\t01\r\n      2146  18F108A7   00000004    8        F0\t00\t00\tFF\tFF\tFF\tFF\t42\r\n      2145  18F106A7   00000004    8        00\tF7\tFF\tFF\tFF\tFF\tFF\t9B\r\n      2145  0CF104A7   00000004    8        F0\t60\t22\tFC\tFF\tFF\tFF\t4D\r\n      2144  0CF103A7   00000004    8        17\t1F\t08\t60\tB1\t1F\t08\t4D\r\n      2172  1FFFFFFF   00000004    8        00\t00\tFF\tFF\tFF\tFF\tFF\tFF\r\n      2163  0CF102A7   00000004    8        30\t75\tE0\t2E\t80\tFF\tFF\tFD\r\n      2163  0CF101A7   00000004    8        68\t00\t97\tCC\t00\t16\t39\t86\r\n      2162  1FFFFFFF   00000004    8        00\t00\tFF\tFF\tFF\tFF\tFF\tFF\r\n      2152  1FFFFFFF   00000004    8        00\t00\tFF\tFF\tFF\tFF\tFF\tFF\r\n      2148  1FFFFFFF   00000004    8        00\t00\tFF\tFF\tFF\tFF\tFF\tFF\r\n      2147  18FEF117   00000004    8        F7\t97\tCC\tCF\tFF\tFF\tFF\tFF\r\n      2146  18F121F0   00000004    8        09\t19\t00\t00\tFF\tFF\tB0\t01\r\n      2146  18F108A7   00000004    8        F0\t00\t00\tFF\tFF\tFF\tFF\t42\r\n      2145  18F106A7   00000004    8        00\tF7\tFF\tFF\tFF\tFF\tFF\t9B\r\n      2145  0CF104A7   00000004    8        F0\t60\t22\tFC\tFF\tFF\tFF\t4D\r\n      2182  1FFFFFFF   00000004    8        00\t00\tFF\tFF\tFF\tFF\tFF\tFF\r\n      2172  1FFFFFFF   00000004    8        00\t00\tFF\tFF\tFF\tFF\tFF\tFF\r\n      2163  0CF102A7   00000004    8        30\t75\tE0\t2E\t80\tFF\tFF\tFD\r\n      2163  0CF101A7   00000004    8        68\t00\t97\tCC\t00\t16\t39\t86\r\n      2162  1FFFFFFF   00000004    8        00\t00\tFF\tFF\tFF\tFF\tFF\tFF\r\n      2152  1FFFFFFF   00000004    8        00\t00\tFF\tFF\tFF\tFF\tFF\tFF\r\n      2148  1FFFFFFF   00000004    8        00\t00\tFF\tFF\tFF\tFF\tFF\tFF\r\n      2147  18FEF117   00000004    8        F7\t97\tCC\tCF\tFF\tFF\tFF\tFF\r\n      2146  18F121F0   00000004    8        09\t19\t00\t00\tFF\tFF\tB0\t01\r\n      2146  18F108A7   00000004    8        F0\t00\t00\tFF\tFF\tFF\tFF\t42\r\n      2145  18F106A7   00000004    8        00\tF7\tFF\tFF\tFF\tFF\tFF\t9B\r\n      2183  0CF101A7   00000004    8        68\t00\t97\tCC\t00\t16\t39\t87\r\n      2182  1FFFFFFF   00000004    8        00\t00\tFF\tFF\tFF\tFF\tFF\tFF\r\n      2172  1FFFFFFF   00000004    8        00\t00\tFF\tFF\tFF\tFF\tFF\tFF\r\n      2163  0CF102A7   00000004    8        30\t75\tE0\t2E\t80\tFF\tFF\tFD\r\n      2163  0CF101A7   00000004    8        68\t00\t97\tCC\t00\t16\t39\t86\r\n      2162  1FFFFFFF   00000004    8        00\t00\tFF\tFF\tFF\tFF\tFF\tFF\r\n      2152  1FFFFFFF   00000004    8        00\t00\tFF\tFF\tFF\tFF\tFF\tFF\r\n      2148  1FFFFFFF   00000004    8        00\t00\tFF\tFF\tFF\tFF\tFF\tFF\r\n      2147  18FEF117   00000004    8        F7\t97\tCC\tCF\tFF\tFF\tFF\tFF\r\n      2146  18F121F0   00000004    8        09\t19\t00\t00\tFF\tFF\tB0\t01\r\n      2146  18F108A7   00000004    8        F0\t00\t00\tFF\tFF\tFF\tFF\t42\r\n      2183  0CF102A7   00000004    8        30\t75\tE0\t2E\t80\tFF\tFF\tFD\r\n      2183  0CF101A7   00000004    8        68\t00\t97\tCC\t00\t16\t39\t87\r\n      2182  1FFFFFFF   00000004    8        00\t00\tFF\tFF\tFF\tFF\tFF\tFF\r\n      2172  1FFFFFFF   00000004    8        00\t00\tFF\tFF\tFF\tFF\tFF\tFF\r\n      2163  0CF102A7   00000004    8        30\t75\tE0\t2E\t80\tFF\tFF\tFD\r\n      2163  0CF101A7   00000004    8        68\t00\t97\tCC\t00\t16\t39\t86\r\n      2162  1FFFFFFF   00000004    8        00\t00\tFF\tFF\tFF\tFF\tFF\tFF\r\n      2152  1FFFFFFF   00000004    8        00\t00\tFF\tFF\tFF\tFF\tFF\tFF\r\n      2148  1FFFFFFF   00000004    8        00\t00\tFF\tFF\tFF\tFF\tFF\tFF\r\n      2147  18FEF117   00000004    8        F7\t97\tCC\tCF\tFF\tFF\tFF\tFF\r\n      2146  18F121F0   00000004    8        09\t19\t00\t00\tFF\tFF\tB0\t01\r\n      2192  1FFFFFFF   00000004    8        00\t00\tFF\tFF\tFF\tFF\tFF\tFF\r\n      2183  0CF102A7   00000004    8        30\t75\tE0\t2E\t80\tFF\tFF\tFD\r\n      2183  0CF101A7   00000004    8        68\t00\t97\tCC\t00\t16\t39\t87\r\n      2182  1FFFFFFF   00000004    8        00\t00\tFF\tFF\tFF\tFF\tFF\tFF\r\n      2172  1FFFFFFF   00000004    8        00\t00\tFF\tFF\tFF\tFF\tFF\tFF\r\n      2163  0CF102A7   00000004    8        30\t75\tE0\t2E\t80\tFF\tFF\tFD\r\n      2163  0CF101A7   00000004    8        68\t00\t97\tCC\t00\t16\t39\t86\r\n      2162  1FFFFFFF   00000004    8        00\t00\tFF\tFF\tFF\tFF\tFF\tFF\r\n      2152  1FFFFFFF   00000004    8        00\t00\tFF\tFF\tFF\tFF\tFF\tFF\r\n      2148  1FFFFFFF   00000004    8        00\t00\tFF\tFF\tFF\tFF\tFF\tFF\r\n      2147  18FEF117   00000004    8        F7\t97\tCC\tCF\tFF\tFF\tFF\tFF\r\n      2193  18F106A7   00000004    8        00\tF7\tFF\tFF\tFF\tFF\tFF\t9C\r\n      2192  1FFFFFFF   00000004    8        00\t00\tFF\tFF\tFF\tFF\tFF\tFF\r\n      2183  0CF102A7   00000004    8        30\t75\tE0\t2E\t80\tFF\tFF\tFD\r\n      2183  0CF101A7   00000004    8        68\t00\t97\tCC\t00\t16\t39\t87\r\n      2182  1FFFFFFF   00000004    8        00\t00\tFF\tFF\tFF\tFF\tFF\tFF\r\n      2172  1FFFFFFF   00000004    8        00\t00\tFF\tFF\tFF\tFF\tFF\tFF\r\n      2163  0CF102A7   00000004    8        30\t75\tE0\t2E\t80\tFF\tFF\tFD\r\n      2163  0CF101A7   00000004    8        68\t00\t97\tCC\t00\t16\t39\t86\r\n      2162  1FFFFFFF   00000004    8        00\t00\tFF\tFF\tFF\tFF\tFF\tFF\r\n      2152  1FFFFFFF   00000004    8        00\t00\tFF\tFF\tFF\tFF\tFF\tFF\r\n      2148  1FFFFFFF   00000004    8        00\t00\tFF\tFF\tFF\tFF\tFF\tFF\r\n      2202  1FFFFFFF   00000004    8        00\t00\tFF\tFF\tFF\tFF\tFF\tFF\r\n      2193  18F106A7   00000004    8        00\tF7\tFF\tFF\tFF\tFF\tFF\t9C\r\n      2192  1FFFFFFF   00000004    8        00\t00\tFF\tFF\tFF\tFF\tFF\tFF\r\n      2183  0CF102A7   00000004    8        30\t75\tE0\t2E\t80\tFF\tFF\tFD\r\n      2183  0CF101A7   00000004    8        68\t00\t97\tCC\t00\t16\t39\t87\r\n      2182  1FFFFFFF   00000004    8        00\t00\tFF\tFF\tFF\tFF\tFF\tFF\r\n      2172  1FFFFFFF   00000004    8        00\t00\tFF\tFF\tFF\tFF\tFF\tFF\r\n      2163  0CF102A7   00000004    8        30\t75\tE0\t2E\t80\tFF\tFF\tFD\r\n      2163  0CF101A7   00000004    8        68\t00\t97\tCC\t00\t16\t39\t86\r\n      2162  1FFFFFFF   00000004    8        00\t00\tFF\tFF\tFF\tFF\tFF\tFF\r\n      2152  1FFFFFFF   00000004    8        00\t00\tFF\tFF\tFF\tFF\tFF\tFF\r\n      2203  0CF101A7   00000004    8        68\t00\t97\tCC\t00\t16\t39\t88\r\n      2202  1FFFFFFF   00000004    8        00\t00\tFF\tFF\tFF\tFF\tFF\tFF\r\n      2193  18F106A7   00000004    8        00\tF7\tFF\tFF\tFF\tFF\tFF\t9C\r\n      2192  1FFFFFFF   00000004    8        00\t00\tFF\tFF\tFF\tFF\tFF\tFF\r\n      2183  0CF102A7   00000004    8        30\t75\tE0\t2E\t80\tFF\tFF\tFD\r\n      2183  0CF101A7   00000004    8        68\t00\t97\tCC\t00\t16\t39\t87\r\n      2182  1FFFFFFF   00000004    8        00\t00\tFF\tFF\tFF\tFF\tFF\tFF\r\n      2172  1FFFFFFF   00000004    8        00\t00\tFF\tFF\tFF\tFF\tFF\tFF\r\n      2163  0CF102A7   00000004    8        30\t75\tE0\t2E\t80\tFF\tFF\tFD\r\n      2163  0CF101A7   00000004    8        68\t00\t97\tCC\t00\t16\t39\t86\r\n      2162  1FFFFFFF   00000004    8        00\t00\tFF\tFF\tFF\tFF\tFF\tFF\r\n      2203  0CF102A7   00000004    8        30\t75\tE0\t2E\t80\tFF\tFF\tFD\r\n      2203  0CF101A7   00000004    8        68\t00\t97\tCC\t00\t16\t39\t88\r\n      2202  1FFFFFFF   00000004    8        00\t00\tFF\tFF\tFF\tFF\tFF\tFF\r\n      2193  18F106A7   00000004    8        00\tF7\tFF\tFF\tFF\tFF\tFF\t9C\r\n      2192  1FFFFFFF   00000004    8        00\t00\tFF\tFF\tFF\tFF\tFF\tFF\r\n      2183  0CF102A7   00000004    8        30\t75\tE0\t2E\t80\tFF\tFF\tFD\r\n      2183  0CF101A7   00000004    8        68\t00\t97\tCC\t00\t16\t39\t87\r\n      2182  1FFFFFFF   00000004    8        00\t00\tFF\tFF\tFF\tFF\tFF\tFF\r\n      2172  1FFFFFFF   00000004    8        00\t00\tFF\tFF\tFF\tFF\tFF\tFF\r\n      2163  0CF102A7   00000004    8        30\t75\tE0\t2E\t80\tFF\tFF\tFD\r\n      2163  0CF101A7   00000004    8        68\t00\t97\tCC\t00\t16\t39\t86\r\n      2212  1FFFFFFF   00000004    8        00\t20\tFF\tFF\tFF\tFF\tFF\tFF\r\n      2203  0CF102A7   00000004    8        30\t75\tE0\t2E\t80\tFF\tFF\tFD\r\n      2203  0CF101A7   00000004    8        68\t00\t97\tCC\t00\t16\t39\t88\r\n      2202  1FFFFFFF   00000004    8        00\t00\tFF\tFF\tFF\tFF\tFF\tFF\r\n      2193  18F106A7   00000004    8        00\tF7\tFF\tFF\tFF\tFF\tFF\t9C\r\n      2192  1FFFFFFF   00000004    8        00\t00\tFF\tFF\tFF\tFF\tFF\tFF\r\n      2183  0CF102A7   00000004    8        30\t75\tE0\t2E\t80\tFF\tFF\tFD\r\n      2183  0CF101A7   00000004    8        68\t00\t97\tCC\t00\t16\t39\t87\r\n      2182  1FFFFFFF   00000004    8        00\t00\tFF\tFF\tFF\tFF\tFF\tFF\r\n      2172  1FFFFFFF   00000004    8        00\t00\tFF\tFF\tFF\tFF\tFF\tFF\r\n      2163  0CF102A7   00000004    8        30\t75\tE0\t2E\t80\tFF\tFF\tFD\r\n      2222  1FFFFFFF   00000004    8        00\t00\tFF\tFF\tFF\tFF\tFF\tFF\r\n      2212  1FFFFFFF   00000004    8        00\t20\tFF\tFF\tFF\tFF\tFF\tFF\r\n      2203  0CF102A7   00000004    8        30\t75\tE0\t2E\t80\tFF\tFF\tFD\r\n      2203  0CF101A7   00000004    8        68\t00\t97\tCC\t00\t
